vi "2022-TestCodeOnTarget.vi"() -> ()   [LabVIEW 2020]
doc: "This VI is called when test mode begins, and will automatically be terminated when it ends. You can add manual or automatic tests and invoke them from the dashboard."
uses:
  <vilib>/Rock Robotics/WPI/ThirdParty/REV Robotics/REVLib/Typedef/Spark MAX Control Type.ctl
  <vilib>/Rock Robotics/WPI/Utilities/WPI_GetSetVariantRefNum.vi
  2022 Robot Global Data.vi
panel:
  out "Error\n(armSetpoint -\n armPosition)":dbl
  out "Commanded\nSet Output":dbl
  out "Premove\nSensor Position":dbl
  out "Sensor Position 2":dbl
  out "armSetpoint":dbl
  out "Sensor Position":dbl
  out "x*y":dbl
  out "element":dbl
  out "x-y":dbl
  out "coerced(x) 2":dbl
  out "coerced(x)":dbl
  out "Position Error 2":dbl
  out "Position Error":dbl
  in  "PID Zero Constants":T1
  out "Status Plot":dbl[](graph)
  out "YRPHfH":T2
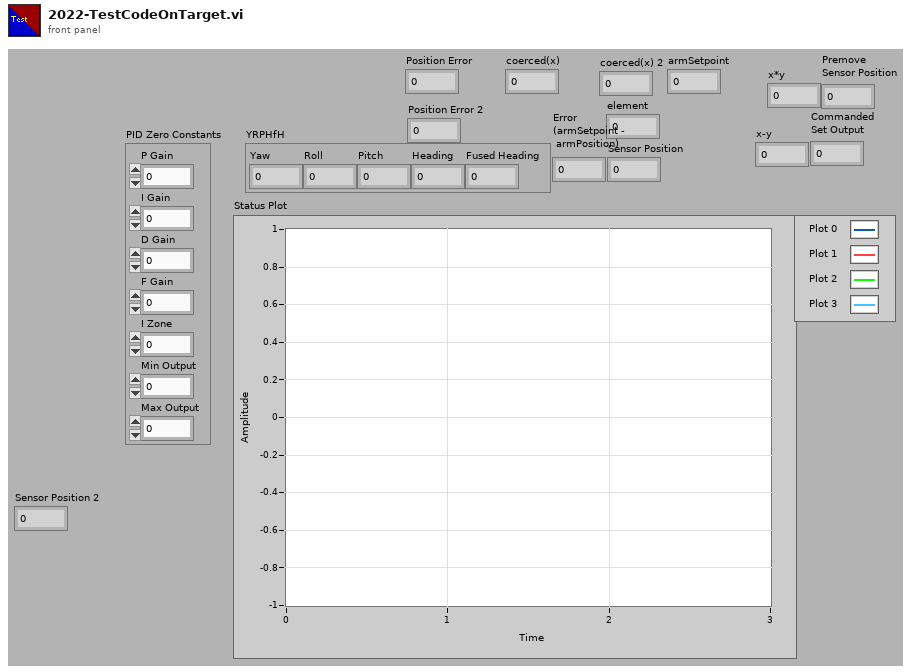
[diagram p1: front panel]
types:
  T1 = cluster{"P Gain":dbl, "I Gain":dbl, "D Gain":dbl, "F Gain":dbl, "I Zone":dbl, "Min Output":dbl, "Max Output":dbl}
  T2 = cluster{"Yaw":dbl, "Roll":dbl, "Pitch":dbl, "Heading":dbl, "Fused Heading":dbl}
  T3 = typedef "WPI_JoystickDevRef.ctl" = cluster{"Device":T4}
  T4 = typedef "WPI_JoystickDeviceEnum.ctl" = enum16{"USB 0", "USB 1", "USB 2", "USB 3", "USB 4", "USB 5"}
  T5 = typedef "WPI_MotorControlDeviceRef.ctl" = cluster{"DeviceStatus":errorcluster, "Type":T6, "PWM":cluster{"PWM Channel":T7, "DeadBand":T8}, "CAN":cluster{"Device Number":u8, "SetOutput VI Ref":variant, "GetOutput VI Ref":variant, "Enable VI Ref":variant, "Disable VI Ref":variant, "Data":variant}, "Invert":bool, "DIO PWM":cluster{"PWM \"Enable\" Channel":T7, "DIOChannel":T9, "PWM Rate":dbl}}
  T6 = typedef "WPI_MotorControlType.ctl" = enum16{"PWM", "CAN", "DIO PWM"}
  T7 = typedef "FPGA_DIOPWMChannel.ctl" = enum8{"PWM 0", "PWM 1", "PWM 2", "PWM 3", "PWM 4", "PWM 5", "PWM 6", "PWM 7", "PWM 8", "PWM 9", "PWM MXP 0", "PWM MXP 1", "PWM MXP 2", "PWM MXP 3", "PWM MXP 4", "PWM MXP 5", "PWM MXP 6", "PWM MXP 7", "PWM MXP 8", "PWM MXP 9", "Invalid"}
  T8 = typedef "WPI_PWMDeadband.ctl" = cluster{"Name":string, "maxPositivePwm":i32, "minPositivePwm":i32, "centerPwm":i32, "maxNegativePwm":i32, "minNegativePwm":i32, "angularRange":u16}
  T9 = typedef "FPGA_DIOChannel.ctl" = enum8{"DIO 0", "DIO 1", "DIO 2", "DIO 3", "DIO 4", "DIO 5", "DIO 6", "DIO 7", "DIO 8", "DIO 9", "DIO MXP 0", "DIO MXP 1", "DIO MXP 2", "DIO MXP 3", "DIO MXP 4", "DIO MXP 5", "DIO MXP 6", "DIO MXP 7", "DIO MXP 8", "DIO MXP 9", "DIO MXP 10", "DIO MXP 11", "DIO MXP 12", "DIO MXP 13", "DIO MXP 14", "DIO MXP 15", "SPI Port CS1", "SPI Port CS2", "SPI Port CS3", "SPI Port MISO", "SPI Port MOSI", "Invalid"}
  T10 = typedef "Spark MAX Control Type.ctl" = enum16{"Percent VBus", "Voltage", "Velocity", "Position", "Smart Motion", "Current", "Smart Velocity"}
  T11 = cluster{"P Gain":bool, "I Gain":bool, "D Gain":bool, "F Gain":bool, "I Zone":bool, "Min Output":bool, "Max Output":bool}
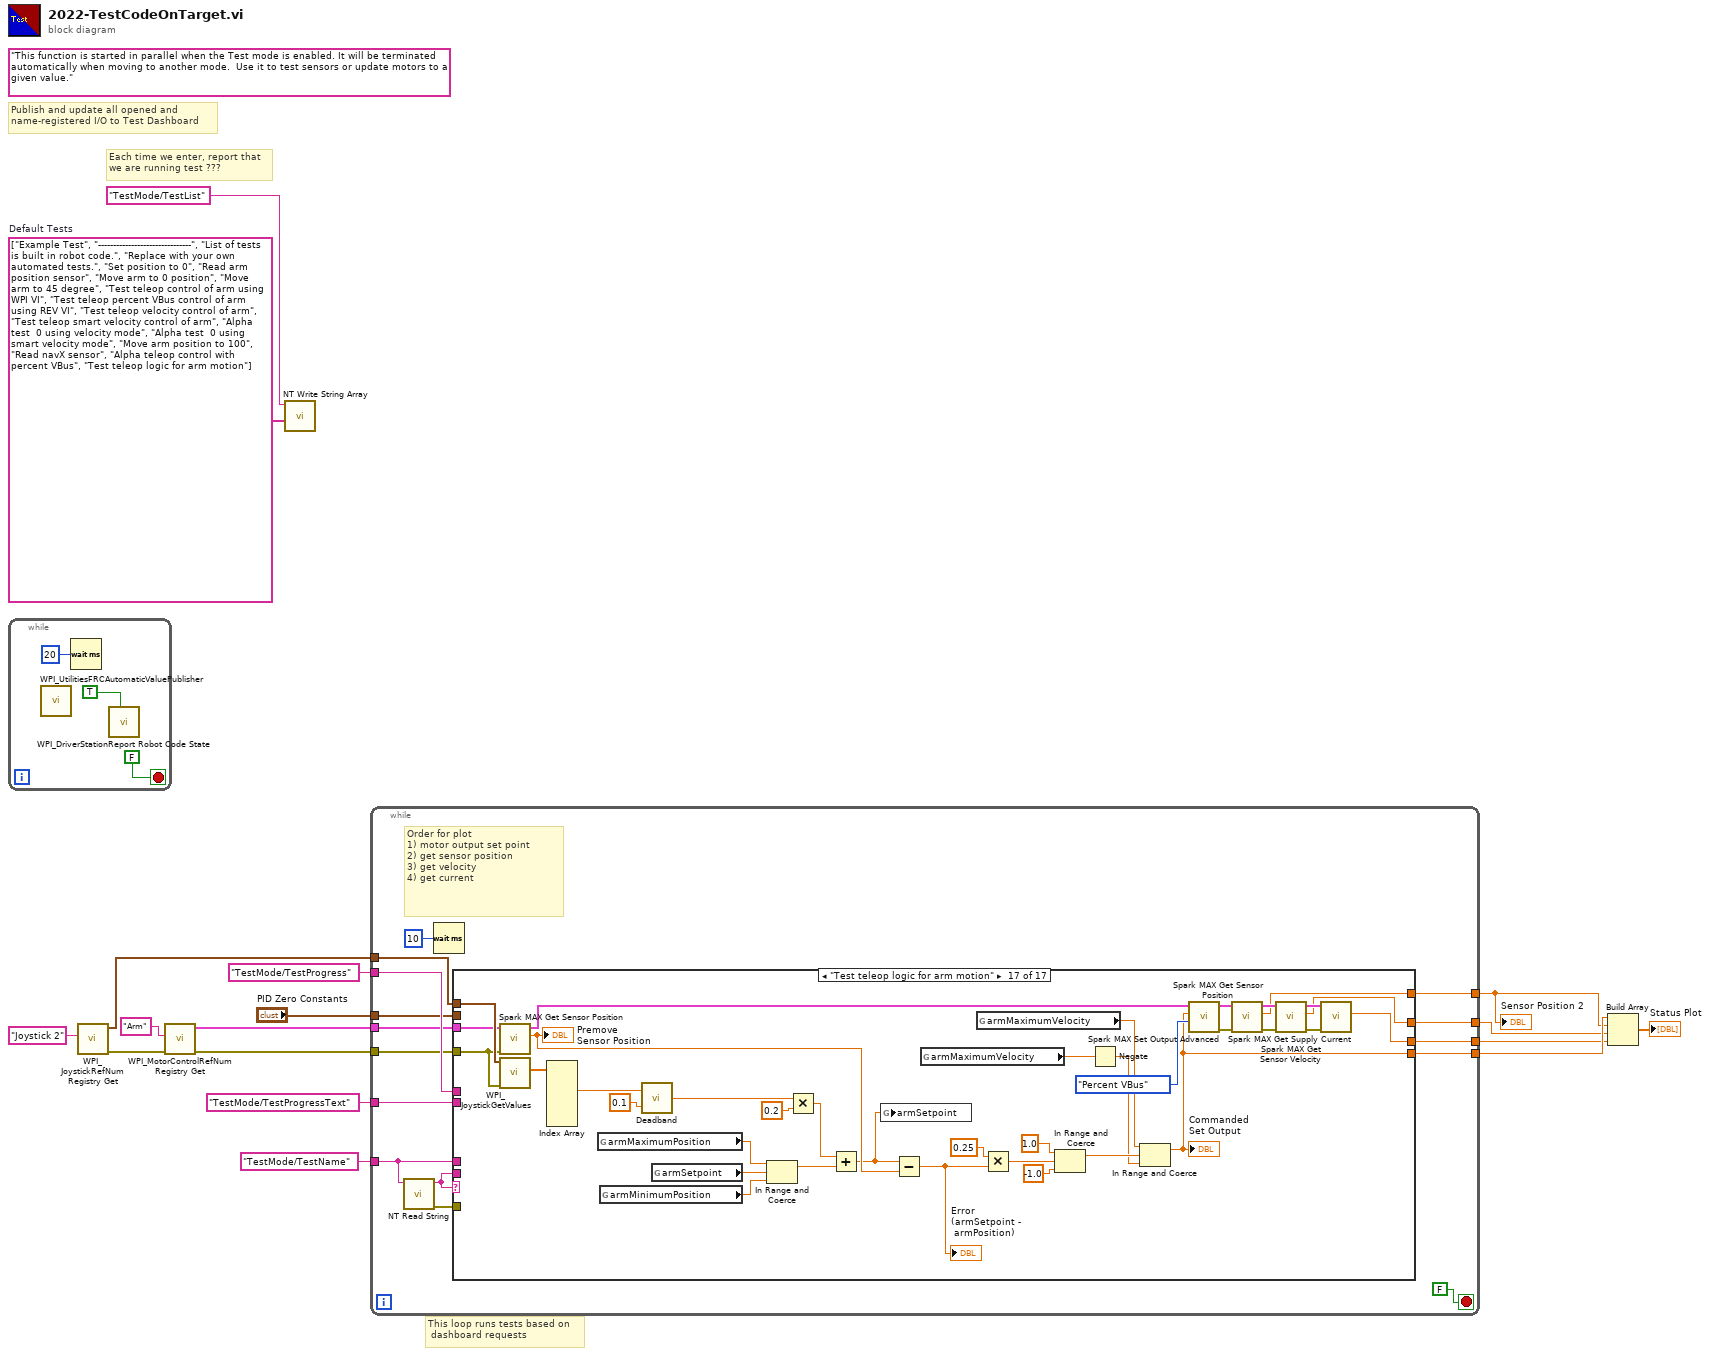
[diagram p0: block diagram]
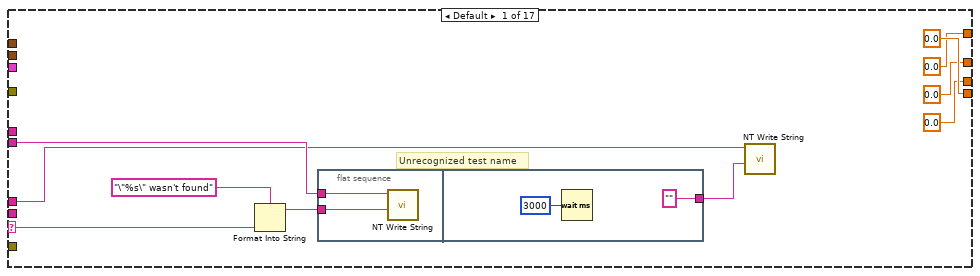
[diagram p2: hidden frame]
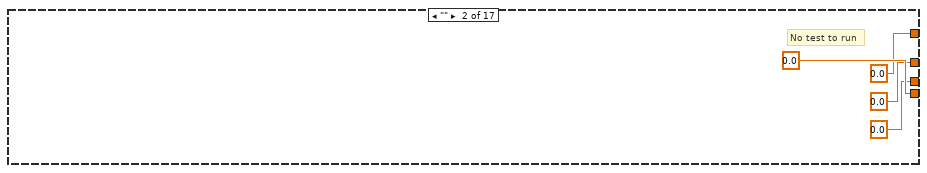
[diagram p3: hidden frame]
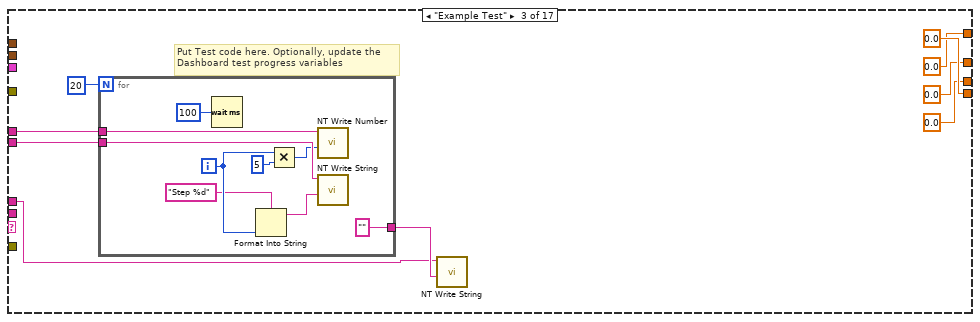
[diagram p4: hidden frame]
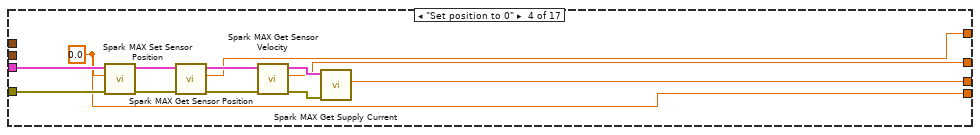
[diagram p5: hidden frame]
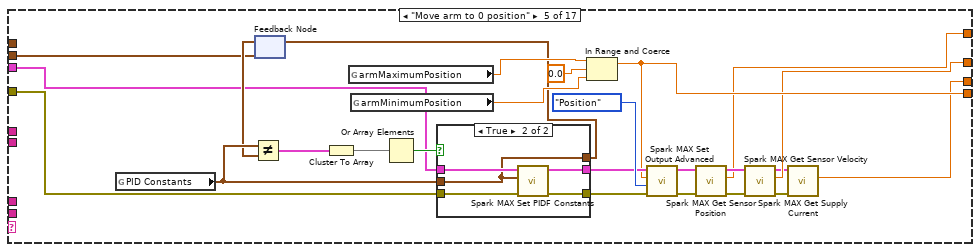
[diagram p6: hidden frame]
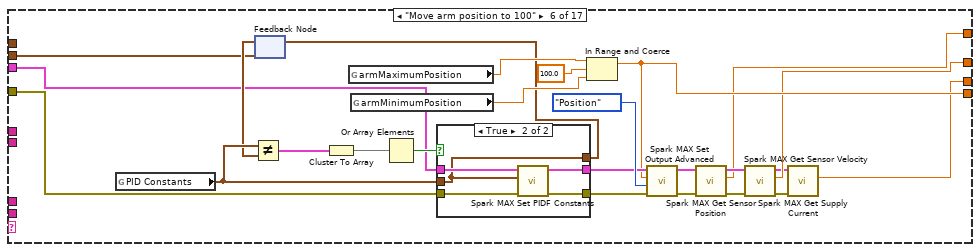
[diagram p8: hidden frame]
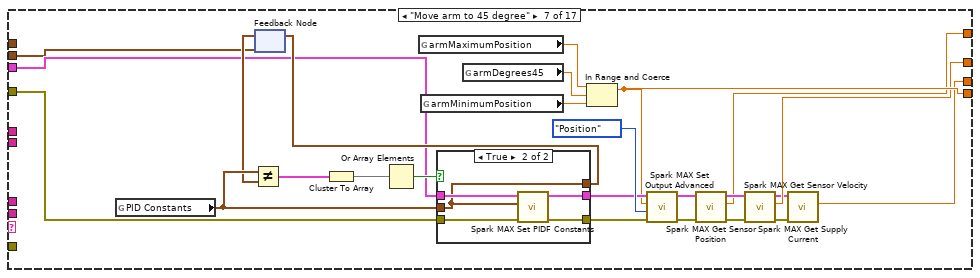
[diagram p10: hidden frame]
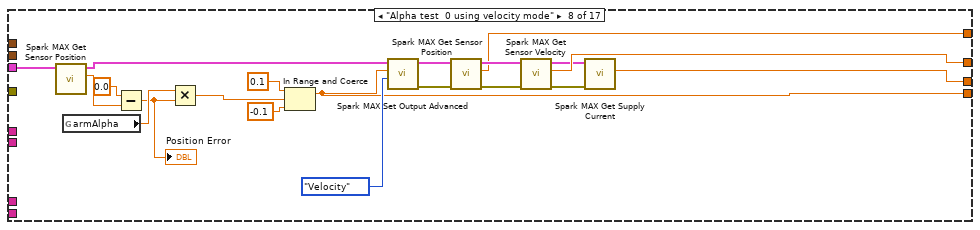
[diagram p12: hidden frame]
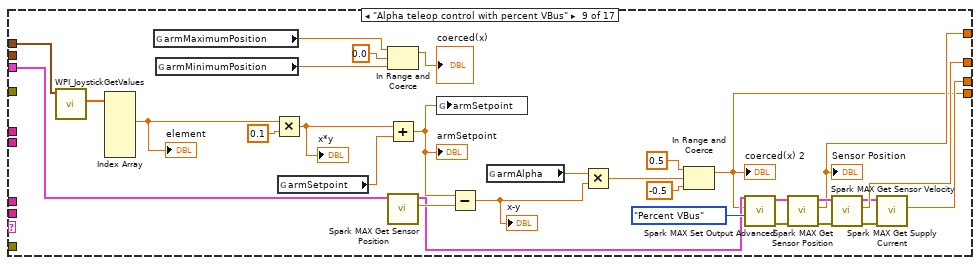
[diagram p13: hidden frame]
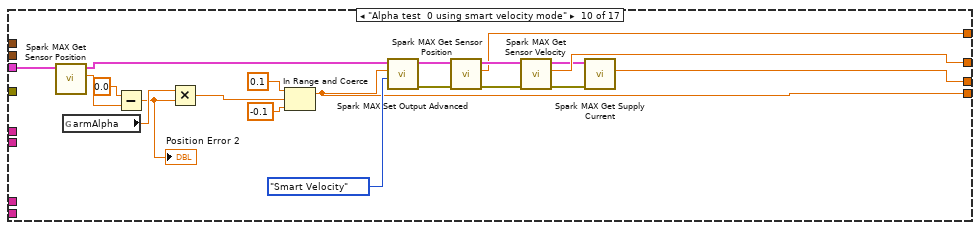
[diagram p14: hidden frame]
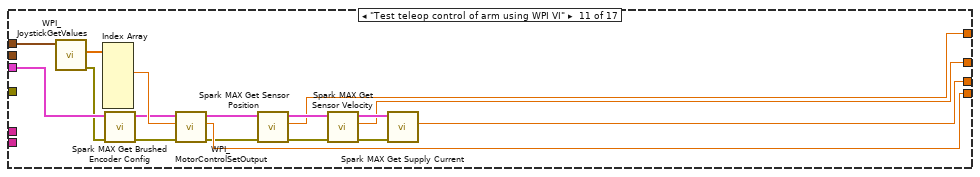
[diagram p15: hidden frame]
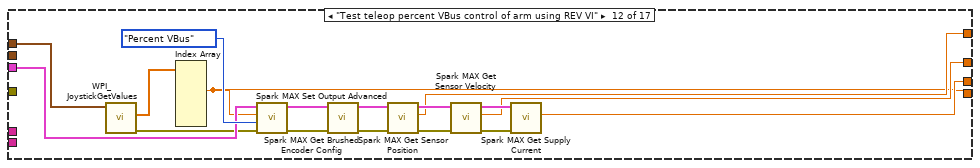
[diagram p16: hidden frame]
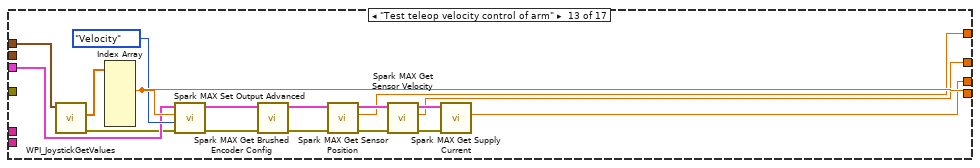
[diagram p17: hidden frame]
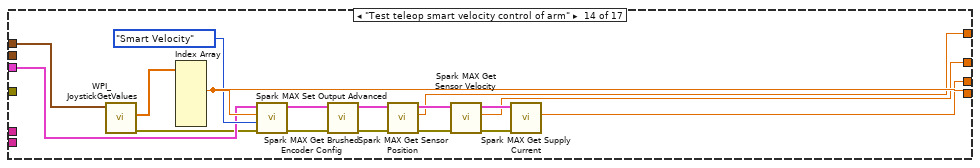
[diagram p18: hidden frame]
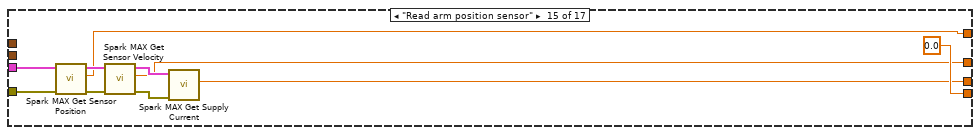
[diagram p19: hidden frame]
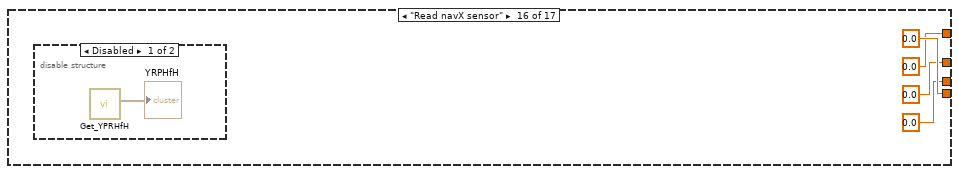
[diagram p20: hidden frame]
diagram:
  w14 = string[] ["Example Test", "-------------------------------", "List of tests is built in robot code.", "Replace with your own automated tests.", "Set position to 0", "Read arm position sensor", "Move arm to 0 position", "Move arm to 45 degree", "Test teleop control of arm using WPI VI", "Test teleop percent VBus control of arm using REV VI", "Test teleop velocity control of arm", "Test teleop smart velocity control of arm", "Alpha test  0 using velocity mode", "Alpha test  0 using smart velocity mode", "Move arm position to 100", "Read navX sensor", "Alpha teleop control with percent VBus", "Test teleop logic for arm motion"]  # Default Tests
  (unwired) "This function is started in parallel when the Test mode is enabled. It will be terminated automatically when moving to another mode.  Use it to test sensors or update motors to a given value."
  # "This loop runs tests based on \n dashboard requests"
  # "Publish and update all opened and\nname-registered I/O to Test Dashboard"
  # "Each time we enter, report that\nwe are running test ???"
  n1 = while {
    stop <- FALSE stop-if-true
    n2 = call <vilib>:"WPI_UtilitiesFRCAutomaticValuePublisher.vi"() -> ()  [unwired: 12 in]
    n3 = Wait (ms)(milliseconds to wait=u32 20) -> ()  [unwired: 1 out]
    n4 = call <vilib>:"WPI_DriverStationReport Robot Code State.vi"("Test"=TRUE ("Autonomous")) -> ()  [unwired: 10 in, 1 out]
  }
  n5 = call <vilib>:"WPI_JoystickRefNum Registry Get.vi"("refnum name"="Joystick 2") -> ("error out"=w1:errorcluster, "JoystickDevRef"=w7:T3)  [unwired: 1 in, 8 out]
  n6 = call <vilib>:"WPI_MotorControlRefNum Registry Get.vi"("error in (no error)"=w1, "refnum name"="Arm") -> ("error out"=w9:errorcluster, "MotorControlDevRef"=w10:T5)  [unwired: 8 in]
  n7 = call <vilib>:"NT Write String Array.vi"("String Array"=w14, "Name"="TestMode/TestList") -> ()  [unwired: 9 in, 1 out]
  n8 = while {
    tunnel: "TestMode/TestName" ("Name") -> [w30]
    tunnel: "TestMode/TestProgressText" ("Name") -> [w33]
    tunnel: "TestMode/TestProgress" ("Name") -> [w32]
    tunnel: w7 -> [w28]
    tunnel: w10 -> [w27]
    tunnel: w9 -> [w26]
    tunnel: "PID Zero Constants" -> [w25]
    tunnel: [w24] -> w5
    tunnel: [w23] -> w2
    tunnel: [w22] -> w4
    tunnel: [w21] -> w3
    stop <- FALSE stop-if-true
    # "Order for plot\n1) motor output set point\n2) get sensor position\n3) get velocity\n4) get current"
    n9 = call <vilib>:"NT Read String.vi"("Name"=w30) -> ("error out"=w29:errorcluster, "String"=w31:string)  [unwired: 9 in]
    n10 = Wait (ms)(milliseconds to wait=u32 10) -> ()  [unwired: 1 out]
    n11 = case shown="\"Test teleop logic for arm motion\"" w31 {
      selector: w31 -> [w44 _ _ _ _ _ _ _ _ _ _ _ _ _ _ _ _]
      tunnel: w30 -> [w41 _ w58 _ _ _ _ _ _ _ _ _ _ _ _ _ _]
      tunnel: w33 -> [w45 _ w61 _ _ _ _ _ _ _ _ _ _ _ _ _ _]
      tunnel: w32 -> [_ _ w62 _ _ _ _ _ _ _ _ _ _ _ _ _ _]
      tunnel: w31 -> [_ _ _ _ _ _ _ _ _ _ _ _ _ _ _ _ _]
      tunnel: w29 -> [_ _ _ _ _ _ _ _ _ _ _ _ _ _ _ _ _]
      tunnel: [0.0 ("armMaximumPosition") 0.0 ("armMaximumPosition") 0.0 ("armMaximumPosition") w81 w93 w126 w159 w183 w214 w233 w268 w270 w302 w319 0.0 ("armMaximumPosition") 0.0 ("armMaximumPosition") w339] -> w24
      tunnel: [0.0 ("Sensor Position") 0.0 ("Sensor Position") 0.0 ("Sensor Position") w73 w92 w125 w158 w199 w229 w249 w255 w272 w288 w305 w323 0.0 ("Sensor Position") w338] -> w23
      tunnel: [0.0 ("Sensor Velocity") 0.0 ("Sensor Velocity") 0.0 ("Sensor Velocity") w72 w91 w124 w157 w198 w228 w248 w254 w271 w287 w304 w322 0.0 ("Sensor Velocity") w337] -> w22
      tunnel: [0.0 ("Sensor Position") 0.0 ("Sensor Position") 0.0 ("Sensor Position") w80 w87 w120 w153 w195 w225 w245 w253 w279 w295 w312 w321 0.0 ("Sensor Position") w336] -> w21
      tunnel: w28 -> [_ _ _ _ _ _ _ _ w204 _ w266 w282 w298 w315 _ _ w366]
      tunnel: w27 -> [_ _ _ w83 w86 w119 w152 w187 w218 w237 w265 w281 w297 w314 w329 _ w365]
      tunnel: w26 -> [_ _ _ w82 w85 w118 w151 _ _ _ _ _ _ _ w330 _ w364]
      tunnel: w25 -> [_ _ _ _ w84 w117 w150 _ _ _ _ _ _ _ _ _ _]
      frame Default {
        # "Unrecognized test name"
        n12 = Format Into String(format string="\"%s\" wasn't found" ("Name"), w44) -> (resulting string=w43:string)  [unwired: 2 in, 1 out]
        n13 = flat-sequence {
          tunnel: w45 -> [w46]
          tunnel: w43 -> [w47]
          tunnel: ["" ("Name")] -> w40
          frame #0 {
            n14 = call <vilib>:"NT Write String.vi"("String"=w47, "Name"=w46) -> ()  [unwired: 9 in, 1 out]
          }
          frame #1 {
            n15 = Wait (ms)(milliseconds to wait=u32 3000) -> ()  [unwired: 1 out]
          }
        }
        n16 = call <vilib>:"NT Write String.vi"("String"=w40, "Name"=w41) -> ()  [unwired: 9 in, 1 out]
      }
      frame "" {
        # "No test to run"
      }
      frame "Example Test" {
        # "Put Test code here. Optionally, update the\nDashboard test progress variables"
        n17 = for {
          N: 20 -> [_]
          tunnel: w62 -> [w71]
          tunnel: w61 -> [w69]
          tunnel: ["" ("String")] -> w59
          i -> [w66]
          n18 = Wait (ms)(milliseconds to wait=u32 100) -> ()  [unwired: 1 out]
          n19 = Format Into String(format string="Step %d", w66) -> (resulting string=w64:string)  [unwired: 2 in, 1 out]
          n20 = Multiply(x=w66, y=u32 5 ("milliseconds to wait")) -> (x*y=w67:u32)
          n21 = call <vilib>:"NT Write Number.vi"("Numeric"=w67, "Name"=w71) -> ()  [unwired: 9 in, 1 out]
          n22 = call <vilib>:"NT Write String.vi"("String"=w64, "Name"=w69) -> ()  [unwired: 9 in, 1 out]
        }
        n23 = call <vilib>:"NT Write String.vi"("String"=w59, "Name"=w58) -> ()  [unwired: 9 in, 1 out]
      }
      frame "Set position to 0" {
        w81 = 0.0 ("Position")
        n24 = call <vilib>:"Spark MAX Set Sensor Position.vi"("error in"=w82, "Position"=w81, "MotorControlDeviceRef"=w83) -> ("error out"=w79:errorcluster, "MotorControlDeviceRef"=w78:T5)  [unwired: 7 in]
        n25 = call <vilib>:"Spark MAX Get Sensor Position.vi"("error in (no error)"=w79, "MotorControlDevRef in"=w78) -> ("error out"=w77:errorcluster, "Sensor Position"=w73:dbl, "MotorControlDevRef out"=w76:T5)  [unwired: 6 in, 1 out]
        n26 = call <vilib>:"Spark MAX Get Sensor Velocity.vi"("error in (no error)"=w77, "MotorControlDevRef in"=w76) -> ("error out"=w74:errorcluster, "Sensor Velocity"=w72:dbl, "MotorControlDevRef out"=w75:T5)  [unwired: 6 in, 1 out]
        n27 = call <vilib>:"Spark MAX Get Supply Current.vi"("error in (no error)"=w74, "MotorControlDevRef in"=w75) -> ("Current"=w80:dbl)  [unwired: 6 in, 3 out]
      }
      frame "Move arm to 0 position" {
        n28 = global read "2022 Robot Global Data.vi" "PID Constants"() -> (w99:T1)
        n29 = feedback #1(w84) -> (w98:T1)
        n30 = Not Equal?(x=w99, y=w98) -> (x != y?=w97:T11)
        n31 = Cluster To Array(cluster=w97) -> (array=w96:bool[])
        n32 = global read "2022 Robot Global Data.vi" "armMaximumPosition"() -> (w107:dbl)
        n33 = global read "2022 Robot Global Data.vi" "armMinimumPosition"() -> (w106:dbl)
        n34 = Or Array Elements(Boolean array=w96) -> (logical OR=w95:bool)
        n35 = case shown="True" w95 {
          tunnel: w85 -> [w109 w116]
          tunnel: w86 -> [w110 w115]
          tunnel: [w109 w114] -> w101
          tunnel: [w110 w113] -> w100
          tunnel: w99 -> [w111 w112]
          tunnel: [w111 w112] -> w94
          frame False {
          }
          frame True {
            n36 = call <vilib>:"Spark MAX Set PIDF Constants.vi"("error in"=w116, "PID Constants"=w112, "MotorControlDeviceRef"=w115) -> ("error out"=w114:errorcluster, "MotorControlDeviceRef"=w113:T5)  [unwired: 7 in]
          }
        }
        n37 = feedback-in #1(w94) -> ()
        n38 = In Range and Coerce(upper limit=w107, x=0.0, lower limit=w106) -> (coerced(x)=w93:dbl)  [unwired: 1 out]
        n39 = call <vilib>:"Spark MAX Set Output Advanced.vi"("error in (no error)"=w101, "Control Mode"=Spark_MAX_Control_Type."Position", "Setpoint"=w93, "MotorControlDevRef"=w100) -> ("error out"=w105:errorcluster, "MotorControlDevRef"=w103:T5)  [unwired: 6 in]
        n40 = call <vilib>:"Spark MAX Get Sensor Position.vi"("error in (no error)"=w105, "MotorControlDevRef in"=w103) -> ("error out"=w104:errorcluster, "Sensor Position"=w92:dbl, "MotorControlDevRef out"=w102:T5)  [unwired: 6 in, 1 out]
        n41 = call <vilib>:"Spark MAX Get Sensor Velocity.vi"("error in (no error)"=w104, "MotorControlDevRef in"=w102) -> ("error out"=w88:errorcluster, "Sensor Velocity"=w91:dbl, "MotorControlDevRef out"=w89:T5)  [unwired: 6 in, 1 out]
        n42 = call <vilib>:"Spark MAX Get Supply Current.vi"("error in (no error)"=w88, "MotorControlDevRef in"=w89) -> ("Current"=w87:dbl)  [unwired: 6 in, 3 out]
      }
      frame "Move arm position to 100" {
        n43 = global read "2022 Robot Global Data.vi" "PID Constants"() -> (w132:T1)
        n44 = feedback #2(w117) -> (w131:T1)
        n45 = Not Equal?(x=w132, y=w131) -> (x != y?=w130:T11)
        n46 = Cluster To Array(cluster=w130) -> (array=w129:bool[])
        n47 = global read "2022 Robot Global Data.vi" "armMaximumPosition"() -> (w140:dbl)
        n48 = global read "2022 Robot Global Data.vi" "armMinimumPosition"() -> (w139:dbl)
        n49 = Or Array Elements(Boolean array=w129) -> (logical OR=w128:bool)
        n50 = case shown="True" w128 {
          tunnel: w118 -> [w142 w149]
          tunnel: w119 -> [w143 w148]
          tunnel: [w142 w147] -> w134
          tunnel: [w143 w146] -> w133
          tunnel: w132 -> [w144 w145]
          tunnel: [w144 w145] -> w127
          frame False {
          }
          frame True {
            n51 = call <vilib>:"Spark MAX Set PIDF Constants.vi"("error in"=w149, "PID Constants"=w145, "MotorControlDeviceRef"=w148) -> ("error out"=w147:errorcluster, "MotorControlDeviceRef"=w146:T5)  [unwired: 7 in]
          }
        }
        n52 = feedback-in #2(w127) -> ()
        n53 = In Range and Coerce(upper limit=w140, x=100.0, lower limit=w139) -> (coerced(x)=w126:dbl)  [unwired: 1 out]
        n54 = call <vilib>:"Spark MAX Set Output Advanced.vi"("error in (no error)"=w134, "Control Mode"=Spark_MAX_Control_Type."Position", "Setpoint"=w126, "MotorControlDevRef"=w133) -> ("error out"=w138:errorcluster, "MotorControlDevRef"=w136:T5)  [unwired: 6 in]
        n55 = call <vilib>:"Spark MAX Get Sensor Position.vi"("error in (no error)"=w138, "MotorControlDevRef in"=w136) -> ("error out"=w137:errorcluster, "Sensor Position"=w125:dbl, "MotorControlDevRef out"=w135:T5)  [unwired: 6 in, 1 out]
        n56 = call <vilib>:"Spark MAX Get Sensor Velocity.vi"("error in (no error)"=w137, "MotorControlDevRef in"=w135) -> ("error out"=w121:errorcluster, "Sensor Velocity"=w124:dbl, "MotorControlDevRef out"=w122:T5)  [unwired: 6 in, 1 out]
        n57 = call <vilib>:"Spark MAX Get Supply Current.vi"("error in (no error)"=w121, "MotorControlDevRef in"=w122) -> ("Current"=w120:dbl)  [unwired: 6 in, 3 out]
      }
      frame "Move arm to 45 degree" {
        n58 = global read "2022 Robot Global Data.vi" "PID Constants"() -> (w164:T1)
        n59 = feedback #3(w150) -> (w163:T1)
        n60 = Not Equal?(x=w164, y=w163) -> (x != y?=w162:T11)
        n61 = Cluster To Array(cluster=w162) -> (array=w161:bool[])
        n62 = Or Array Elements(Boolean array=w161) -> (logical OR=w160:bool)
        n63 = global read "2022 Robot Global Data.vi" "armMaximumPosition"() -> (w173:dbl)
        n64 = global read "2022 Robot Global Data.vi" "armMinimumPosition"() -> (w172:dbl)
        n65 = case shown="True" w160 {
          tunnel: w151 -> [w175 w182]
          tunnel: w152 -> [w176 w181]
          tunnel: [w175 w180] -> w166
          tunnel: [w176 w179] -> w165
          tunnel: w164 -> [w177 w178]
          tunnel: [w177 w178] -> w156
          frame False {
          }
          frame True {
            n66 = call <vilib>:"Spark MAX Set PIDF Constants.vi"("error in"=w182, "PID Constants"=w178, "MotorControlDeviceRef"=w181) -> ("error out"=w180:errorcluster, "MotorControlDeviceRef"=w179:T5)  [unwired: 7 in]
          }
        }
        n67 = feedback-in #3(w156) -> ()
        n68 = global read "2022 Robot Global Data.vi" "armDegrees45"() -> (w171:dbl)
        n69 = In Range and Coerce(upper limit=w173, x=w171, lower limit=w172) -> (coerced(x)=w159:dbl)  [unwired: 1 out]
        n70 = call <vilib>:"Spark MAX Set Output Advanced.vi"("error in (no error)"=w166, "Control Mode"=Spark_MAX_Control_Type."Position", "Setpoint"=w159, "MotorControlDevRef"=w165) -> ("error out"=w170:errorcluster, "MotorControlDevRef"=w168:T5)  [unwired: 6 in]
        n71 = call <vilib>:"Spark MAX Get Sensor Position.vi"("error in (no error)"=w170, "MotorControlDevRef in"=w168) -> ("error out"=w169:errorcluster, "Sensor Position"=w158:dbl, "MotorControlDevRef out"=w167:T5)  [unwired: 6 in, 1 out]
        n72 = call <vilib>:"Spark MAX Get Sensor Velocity.vi"("error in (no error)"=w169, "MotorControlDevRef in"=w167) -> ("error out"=w154:errorcluster, "Sensor Velocity"=w157:dbl, "MotorControlDevRef out"=w155:T5)  [unwired: 6 in, 1 out]
        n73 = call <vilib>:"Spark MAX Get Supply Current.vi"("error in (no error)"=w154, "MotorControlDevRef in"=w155) -> ("Current"=w153:dbl)  [unwired: 6 in, 3 out]
      }
      frame "Alpha test  0 using velocity mode" {
        n74 = call <vilib>:"Spark MAX Get Sensor Position.vi"("MotorControlDevRef in"=w187) -> ("Sensor Position"=w193:dbl, "MotorControlDevRef out"=w186:T5)  [unwired: 7 in, 2 out]
        n75 = global read "2022 Robot Global Data.vi" "armAlpha"() -> (w192:dbl)
        n76 = Subtract(x=0.0, y=w193) -> (x-y=w191:dbl)
        "Position Error" <- w191
        n77 = Multiply(x=w192, y=w191) -> (x*y=w188:dbl)
        n78 = In Range and Coerce(upper limit=0.1, x=w188, lower limit=-0.1) -> (coerced(x)=w183:dbl)  [unwired: 1 out]
        n79 = call <vilib>:"Spark MAX Set Output Advanced.vi"("Control Mode"=Spark_MAX_Control_Type."Velocity", "Setpoint"=w183, "MotorControlDevRef"=w186) -> ("error out"=w184:errorcluster, "MotorControlDevRef"=w185:T5)  [unwired: 7 in]
        n80 = call <vilib>:"Spark MAX Get Sensor Position.vi"("error in (no error)"=w184, "MotorControlDevRef in"=w185) -> ("error out"=w201:errorcluster, "Sensor Position"=w199:dbl, "MotorControlDevRef out"=w200:T5)  [unwired: 6 in, 1 out]
        n81 = call <vilib>:"Spark MAX Get Sensor Velocity.vi"("error in (no error)"=w201, "MotorControlDevRef in"=w200) -> ("error out"=w196:errorcluster, "Sensor Velocity"=w198:dbl, "MotorControlDevRef out"=w197:T5)  [unwired: 6 in, 1 out]
        n82 = call <vilib>:"Spark MAX Get Supply Current.vi"("error in (no error)"=w196, "MotorControlDevRef in"=w197) -> ("Current"=w195:dbl)  [unwired: 6 in, 3 out]
      }
      frame "Alpha teleop control with percent VBus" {
        n83 = call <vilib>:"WPI_JoystickGetValues.vi"("JoystickDevRef"=w204) -> ("Axes"=w210:dbl[])  [unwired: 6 in, 4 out]
        n84 = Index Array(array=w210) -> (element #2=w203:dbl)  [unwired: 6 in, 5 out]
        "element" <- w203
        n85 = global read "2022 Robot Global Data.vi" "armMaximumPosition"() -> (w213:dbl)
        n86 = global read "2022 Robot Global Data.vi" "armMinimumPosition"() -> (w212:dbl)
        n87 = Multiply(x=w203, y=0.1) -> (x*y=w208:dbl)
        "x*y" <- w208
        n88 = global read "2022 Robot Global Data.vi" "armSetpoint"() -> (w207:dbl)
        n89 = In Range and Coerce(upper limit=w213, x=0.0, lower limit=w212) -> (coerced(x)=→"coerced(x)":dbl)  [unwired: 1 out]
        n90 = Add(x=w208, y=w207) -> (x+y=w206:dbl)
        "armSetpoint" <- w206
        n91 = call <vilib>:"Spark MAX Get Sensor Position.vi"("MotorControlDevRef in"=w218) -> ("Sensor Position"=w224:dbl, "MotorControlDevRef out"=w217:T5)  [unwired: 7 in, 2 out]
        n92 = global write "2022 Robot Global Data.vi" "armSetpoint"(w206) -> ()
        n93 = Subtract(x=w206, y=w224) -> (x-y=w222:dbl)
        "x-y" <- w222
        n94 = global read "2022 Robot Global Data.vi" "armAlpha"() -> (w223:dbl)
        n95 = Multiply(x=w223, y=w222) -> (x*y=w219:dbl)
        n96 = In Range and Coerce(upper limit=0.5, x=w219, lower limit=-0.5) -> (coerced(x)=w214:dbl)  [unwired: 1 out]
        "coerced(x) 2" <- w214
        n97 = call <vilib>:"Spark MAX Set Output Advanced.vi"("Control Mode"=Spark_MAX_Control_Type."Percent VBus", "Setpoint"=w214, "MotorControlDevRef"=w217) -> ("error out"=w215:errorcluster, "MotorControlDevRef"=w216:T5)  [unwired: 7 in]
        n98 = call <vilib>:"Spark MAX Get Sensor Position.vi"("error in (no error)"=w215, "MotorControlDevRef in"=w216) -> ("error out"=w231:errorcluster, "Sensor Position"=w229:dbl, "MotorControlDevRef out"=w230:T5)  [unwired: 6 in, 1 out]
        "Sensor Position" <- w229
        n99 = call <vilib>:"Spark MAX Get Sensor Velocity.vi"("error in (no error)"=w231, "MotorControlDevRef in"=w230) -> ("error out"=w226:errorcluster, "Sensor Velocity"=w228:dbl, "MotorControlDevRef out"=w227:T5)  [unwired: 6 in, 1 out]
        n100 = call <vilib>:"Spark MAX Get Supply Current.vi"("error in (no error)"=w226, "MotorControlDevRef in"=w227) -> ("Current"=w225:dbl)  [unwired: 6 in, 3 out]
      }
      frame "Alpha test  0 using smart velocity mode" {
        n101 = call <vilib>:"Spark MAX Get Sensor Position.vi"("MotorControlDevRef in"=w237) -> ("Sensor Position"=w243:dbl, "MotorControlDevRef out"=w236:T5)  [unwired: 7 in, 2 out]
        n102 = global read "2022 Robot Global Data.vi" "armAlpha"() -> (w242:dbl)
        n103 = Subtract(x=0.0, y=w243) -> (x-y=w241:dbl)
        "Position Error 2" <- w241
        n104 = Multiply(x=w242, y=w241) -> (x*y=w238:dbl)
        n105 = In Range and Coerce(upper limit=0.1, x=w238, lower limit=-0.1) -> (coerced(x)=w233:dbl)  [unwired: 1 out]
        n106 = call <vilib>:"Spark MAX Set Output Advanced.vi"("Control Mode"=Spark_MAX_Control_Type."Smart Velocity", "Setpoint"=w233, "MotorControlDevRef"=w236) -> ("error out"=w234:errorcluster, "MotorControlDevRef"=w235:T5)  [unwired: 7 in]
        n107 = call <vilib>:"Spark MAX Get Sensor Position.vi"("error in (no error)"=w234, "MotorControlDevRef in"=w235) -> ("error out"=w251:errorcluster, "Sensor Position"=w249:dbl, "MotorControlDevRef out"=w250:T5)  [unwired: 6 in, 1 out]
        n108 = call <vilib>:"Spark MAX Get Sensor Velocity.vi"("error in (no error)"=w251, "MotorControlDevRef in"=w250) -> ("error out"=w246:errorcluster, "Sensor Velocity"=w248:dbl, "MotorControlDevRef out"=w247:T5)  [unwired: 6 in, 1 out]
        n109 = call <vilib>:"Spark MAX Get Supply Current.vi"("error in (no error)"=w246, "MotorControlDevRef in"=w247) -> ("Current"=w245:dbl)  [unwired: 6 in, 3 out]
      }
      frame "Test teleop control of arm using WPI VI" {
        n110 = call <vilib>:"WPI_JoystickGetValues.vi"("JoystickDevRef"=w266) -> ("error out"=w264:errorcluster, "Axes"=w269:dbl[])  [unwired: 6 in, 3 out]
        n111 = Index Array(array=w269) -> (element #2=w267:dbl)  [unwired: 6 in, 5 out]
        n112 = call <vilib>:"Spark MAX Get Brushed Encoder Config.vi"("error in (no error)"=w264, "MotorControlDeviceRef in"=w265) -> ("error out"=w262:errorcluster, "MotorControlDeviceRef"=w263:T5)  [unwired: 4 in, 4 out]
        n113 = call <vilib>:"WPI_MotorControlSetOutput.vi"("error in (no error)"=w262, "Output"=w267, "MotorControlDevRef"=w263) -> ("error out"=w261:errorcluster, "Motor Output"=w268:dbl, "MotorControlDevRef"=w258:T5)  [unwired: 6 in]
        n114 = call <vilib>:"Spark MAX Get Sensor Position.vi"("error in (no error)"=w261, "MotorControlDevRef in"=w258) -> ("error out"=w260:errorcluster, "Sensor Position"=w255:dbl, "MotorControlDevRef out"=w257:T5)  [unwired: 6 in, 1 out]
        n115 = call <vilib>:"Spark MAX Get Sensor Velocity.vi"("error in (no error)"=w260, "MotorControlDevRef in"=w257) -> ("error out"=w259:errorcluster, "Sensor Velocity"=w254:dbl, "MotorControlDevRef out"=w256:T5)  [unwired: 6 in, 1 out]
        n116 = call <vilib>:"Spark MAX Get Supply Current.vi"("error in (no error)"=w259, "MotorControlDevRef in"=w256) -> ("Current"=w253:dbl)  [unwired: 6 in, 3 out]
      }
      frame "Test teleop percent VBus control of arm using REV VI" {
        n117 = call <vilib>:"WPI_JoystickGetValues.vi"("JoystickDevRef"=w282) -> ("error out"=w280:errorcluster, "Axes"=w286:dbl[])  [unwired: 6 in, 3 out]
        n118 = Index Array(array=w286) -> (element #2=w270:dbl)  [unwired: 6 in, 5 out]
        n119 = call <vilib>:"Spark MAX Set Output Advanced.vi"("error in (no error)"=w280, "Control Mode"=Spark_MAX_Control_Type."Percent VBus", "Setpoint"=w270, "MotorControlDevRef"=w281) -> ("error out"=w283:errorcluster, "MotorControlDevRef"=w284:T5)  [unwired: 6 in]
        n120 = call <vilib>:"Spark MAX Get Brushed Encoder Config.vi"("error in (no error)"=w283, "MotorControlDeviceRef in"=w284) -> ("error out"=w275:errorcluster, "MotorControlDeviceRef"=w278:T5)  [unwired: 4 in, 4 out]
        n121 = call <vilib>:"Spark MAX Get Sensor Position.vi"("error in (no error)"=w275, "MotorControlDevRef in"=w278) -> ("error out"=w274:errorcluster, "Sensor Position"=w272:dbl, "MotorControlDevRef out"=w277:T5)  [unwired: 6 in, 1 out]
        n122 = call <vilib>:"Spark MAX Get Sensor Velocity.vi"("error in (no error)"=w274, "MotorControlDevRef in"=w277) -> ("error out"=w273:errorcluster, "Sensor Velocity"=w271:dbl, "MotorControlDevRef out"=w276:T5)  [unwired: 6 in, 1 out]
        n123 = call <vilib>:"Spark MAX Get Supply Current.vi"("error in (no error)"=w273, "MotorControlDevRef in"=w276) -> ("Current"=w279:dbl)  [unwired: 6 in, 3 out]
      }
      frame "Test teleop velocity control of arm" {
        n124 = call <vilib>:"WPI_JoystickGetValues.vi"("JoystickDevRef"=w298) -> ("error out"=w296:errorcluster, "Axes"=w303:dbl[])  [unwired: 6 in, 3 out]
        n125 = Index Array(array=w303) -> (element #2=w302:dbl)  [unwired: 6 in, 5 out]
        n126 = call <vilib>:"Spark MAX Set Output Advanced.vi"("error in (no error)"=w296, "Control Mode"=Spark_MAX_Control_Type."Velocity", "Setpoint"=w302, "MotorControlDevRef"=w297) -> ("error out"=w299:errorcluster, "MotorControlDevRef"=w300:T5)  [unwired: 6 in]
        n127 = call <vilib>:"Spark MAX Get Brushed Encoder Config.vi"("error in (no error)"=w299, "MotorControlDeviceRef in"=w300) -> ("error out"=w291:errorcluster, "MotorControlDeviceRef"=w294:T5)  [unwired: 4 in, 4 out]
        n128 = call <vilib>:"Spark MAX Get Sensor Position.vi"("error in (no error)"=w291, "MotorControlDevRef in"=w294) -> ("error out"=w290:errorcluster, "Sensor Position"=w288:dbl, "MotorControlDevRef out"=w293:T5)  [unwired: 6 in, 1 out]
        n129 = call <vilib>:"Spark MAX Get Sensor Velocity.vi"("error in (no error)"=w290, "MotorControlDevRef in"=w293) -> ("error out"=w289:errorcluster, "Sensor Velocity"=w287:dbl, "MotorControlDevRef out"=w292:T5)  [unwired: 6 in, 1 out]
        n130 = call <vilib>:"Spark MAX Get Supply Current.vi"("error in (no error)"=w289, "MotorControlDevRef in"=w292) -> ("Current"=w295:dbl)  [unwired: 6 in, 3 out]
      }
      frame "Test teleop smart velocity control of arm" {
        n131 = call <vilib>:"WPI_JoystickGetValues.vi"("JoystickDevRef"=w315) -> ("error out"=w313:errorcluster, "Axes"=w320:dbl[])  [unwired: 6 in, 3 out]
        n132 = Index Array(array=w320) -> (element #2=w319:dbl)  [unwired: 6 in, 5 out]
        n133 = call <vilib>:"Spark MAX Set Output Advanced.vi"("error in (no error)"=w313, "Control Mode"=Spark_MAX_Control_Type."Smart Velocity", "Setpoint"=w319, "MotorControlDevRef"=w314) -> ("error out"=w316:errorcluster, "MotorControlDevRef"=w317:T5)  [unwired: 6 in]
        n134 = call <vilib>:"Spark MAX Get Brushed Encoder Config.vi"("error in (no error)"=w316, "MotorControlDeviceRef in"=w317) -> ("error out"=w308:errorcluster, "MotorControlDeviceRef"=w311:T5)  [unwired: 4 in, 4 out]
        n135 = call <vilib>:"Spark MAX Get Sensor Position.vi"("error in (no error)"=w308, "MotorControlDevRef in"=w311) -> ("error out"=w307:errorcluster, "Sensor Position"=w305:dbl, "MotorControlDevRef out"=w310:T5)  [unwired: 6 in, 1 out]
        n136 = call <vilib>:"Spark MAX Get Sensor Velocity.vi"("error in (no error)"=w307, "MotorControlDevRef in"=w310) -> ("error out"=w306:errorcluster, "Sensor Velocity"=w304:dbl, "MotorControlDevRef out"=w309:T5)  [unwired: 6 in, 1 out]
        n137 = call <vilib>:"Spark MAX Get Supply Current.vi"("error in (no error)"=w306, "MotorControlDevRef in"=w309) -> ("Current"=w312:dbl)  [unwired: 6 in, 3 out]
      }
      frame "Read arm position sensor" {
        n138 = call <vilib>:"Spark MAX Get Sensor Position.vi"("error in (no error)"=w330, "MotorControlDevRef in"=w329) -> ("error out"=w327:errorcluster, "Sensor Position"=w323:dbl, "MotorControlDevRef out"=w328:T5)  [unwired: 6 in, 1 out]
        n139 = call <vilib>:"Spark MAX Get Sensor Velocity.vi"("error in (no error)"=w327, "MotorControlDevRef in"=w328) -> ("error out"=w325:errorcluster, "Sensor Velocity"=w322:dbl, "MotorControlDevRef out"=w326:T5)  [unwired: 6 in, 1 out]
        n140 = call <vilib>:"Spark MAX Get Supply Current.vi"("error in (no error)"=w325, "MotorControlDevRef in"=w326) -> ("Current"=w321:dbl)  [unwired: 6 in, 3 out]
      }
      frame "Read navX sensor" {
        n141 = disable-structure shown="Disabled" {
          frame Disabled {
            n142 = call <vilib>:"Get_YPRHfH.vi"() -> ("YRPHfH"=→"YRPHfH":T2)  [unwired: 11 in]
          }
          frame Enabled {
          }
        }
      }
      frame "Test teleop logic for arm motion" {
        n143 = call <vilib>:"Spark MAX Get Sensor Position.vi"("error in (no error)"=w364, "MotorControlDevRef in"=w365) -> ("Sensor Position"=w353:dbl, "MotorControlDevRef out"=w345:T5)  [unwired: 6 in, 2 out]
        "Premove\nSensor Position" <- w353
        n144 = call <vilib>:"WPI_JoystickGetValues.vi"("error in (no error)"=w364, "JoystickDevRef"=w366) -> ("Axes"=w371:dbl[])  [unwired: 5 in, 4 out]
        n145 = Index Array(array=w371) -> (element #2=w368:dbl)  [unwired: 6 in, 5 out]
        n146 = global read "2022 Robot Global Data.vi" "armMaximumPosition"() -> (w362:dbl)
        n147 = global read "2022 Robot Global Data.vi" "armMinimumPosition"() -> (w363:dbl)
        n148 = call "Deadband.vi"("Limit"=0.1, "Input"=w368) -> ("Output"=w367:dbl)
        n149 = global read "2022 Robot Global Data.vi" "armSetpoint"() -> (w361:dbl)
        n150 = In Range and Coerce(upper limit=w362, x=w361, lower limit=w363) -> (coerced(x)=w359:dbl)  [unwired: 1 out]
        n151 = Multiply(x=w367, y=0.2) -> (x*y=w360:dbl)
        n152 = Add(x=w360, y=w359) -> (x+y=w352:dbl)
        n153 = global write "2022 Robot Global Data.vi" "armSetpoint"(w352) -> ()
        n154 = Subtract(x=w352, y=w353) -> (x-y=w358:dbl)
        "Error\n(armSetpoint -\n armPosition)" <- w358
        n155 = global read "2022 Robot Global Data.vi" "armMaximumVelocity"() -> (w342:dbl)
        n156 = global read "2022 Robot Global Data.vi" "armMaximumVelocity"() -> (w344:dbl)
        n157 = Multiply(x=0.25, y=w358) -> (x*y=w355:dbl)
        n158 = In Range and Coerce(upper limit=1.0, x=w355, lower limit=-1.0) -> (coerced(x)=w343:dbl)  [unwired: 1 out]
        n159 = Negate(x=w342) -> (-x=w341:dbl)
        n160 = In Range and Coerce(upper limit=w344, x=w343, lower limit=w341) -> (coerced(x)=w339:dbl)  [unwired: 1 out]
        "Commanded\nSet Output" <- w339
        n161 = call <vilib>:"Spark MAX Set Output Advanced.vi"("Control Mode"=Spark_MAX_Control_Type."Percent VBus", "Setpoint"=w339, "MotorControlDevRef"=w345) -> ("error out"=w346:errorcluster, "MotorControlDevRef"=w347:T5)  [unwired: 7 in]
        n162 = call <vilib>:"Spark MAX Get Sensor Position.vi"("error in (no error)"=w346, "MotorControlDevRef in"=w347) -> ("error out"=w351:errorcluster, "Sensor Position"=w338:dbl, "MotorControlDevRef out"=w350:T5)  [unwired: 6 in, 1 out]
        n163 = call <vilib>:"Spark MAX Get Sensor Velocity.vi"("error in (no error)"=w351, "MotorControlDevRef in"=w350) -> ("error out"=w348:errorcluster, "Sensor Velocity"=w337:dbl, "MotorControlDevRef out"=w349:T5)  [unwired: 6 in, 1 out]
        n164 = call <vilib>:"Spark MAX Get Supply Current.vi"("error in (no error)"=w348, "MotorControlDevRef in"=w349) -> ("Current"=w336:dbl)  [unwired: 6 in, 3 out]
      }
    }
  }
  "Sensor Position 2" <- w2
  n165 = Build Array(w5, w2, w4, w3) -> (→"Status Plot":dbl[])
